vi "CurrentSweepExample.vi"(4 "Points":i32, 5 "milliseconds to wait":u32=10000, 6 "End Current":dbl=1.0, 7 "Start Current":dbl, 8 "Stanford Err":errorcluster, 9 "Stanford":refnum<visa-resource-name>, 10 "Keithley Err":errorcluster, 11 "Keithley":refnum<visa-resource-name>) -> (0 "Stanford Err Out":errorcluster, 1 "Stanford Out":refnum<visa-resource-name>, 2 "Keithley Err Out":errorcluster, 3 "Keithley Out":refnum<visa-resource-name>)   [LabVIEW 2013]
uses:
  <vilib>/Analysis/1siggen.llb/Ramp Pattern by Samples.vi
  Stop_B_Global.vi
  He3_Tlogger_Global 1.vi
  <vilib>/Analysis/NI_AALBase.lvlib
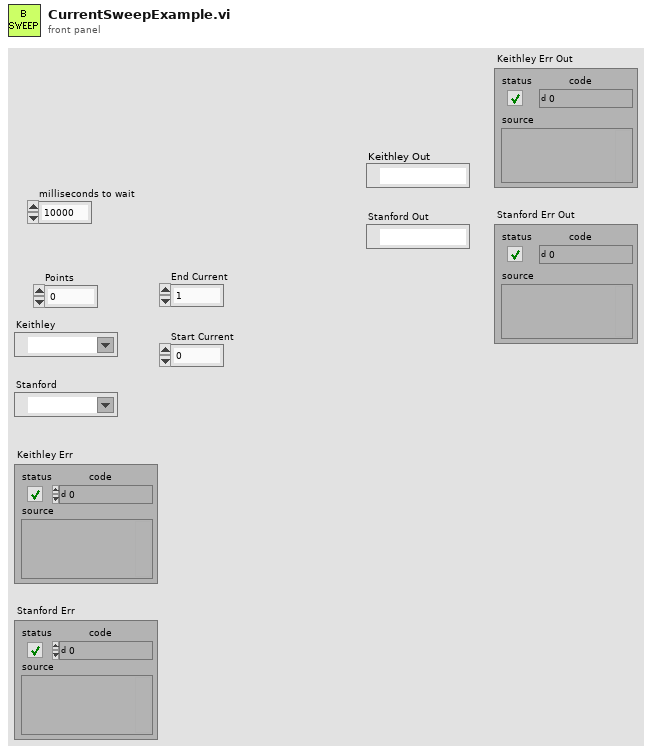
[diagram p1: front panel]
types:
  T1 = cluster{"Stanford Current":dbl, "X-Value":dbl, "Y-Value":dbl, "R-Value":dbl, "Theta-Value":dbl, "Reference Frequency":dbl, "Field":dbl, "Temperature":dbl, "Resistance":dbl, "Integration Time":dbl}
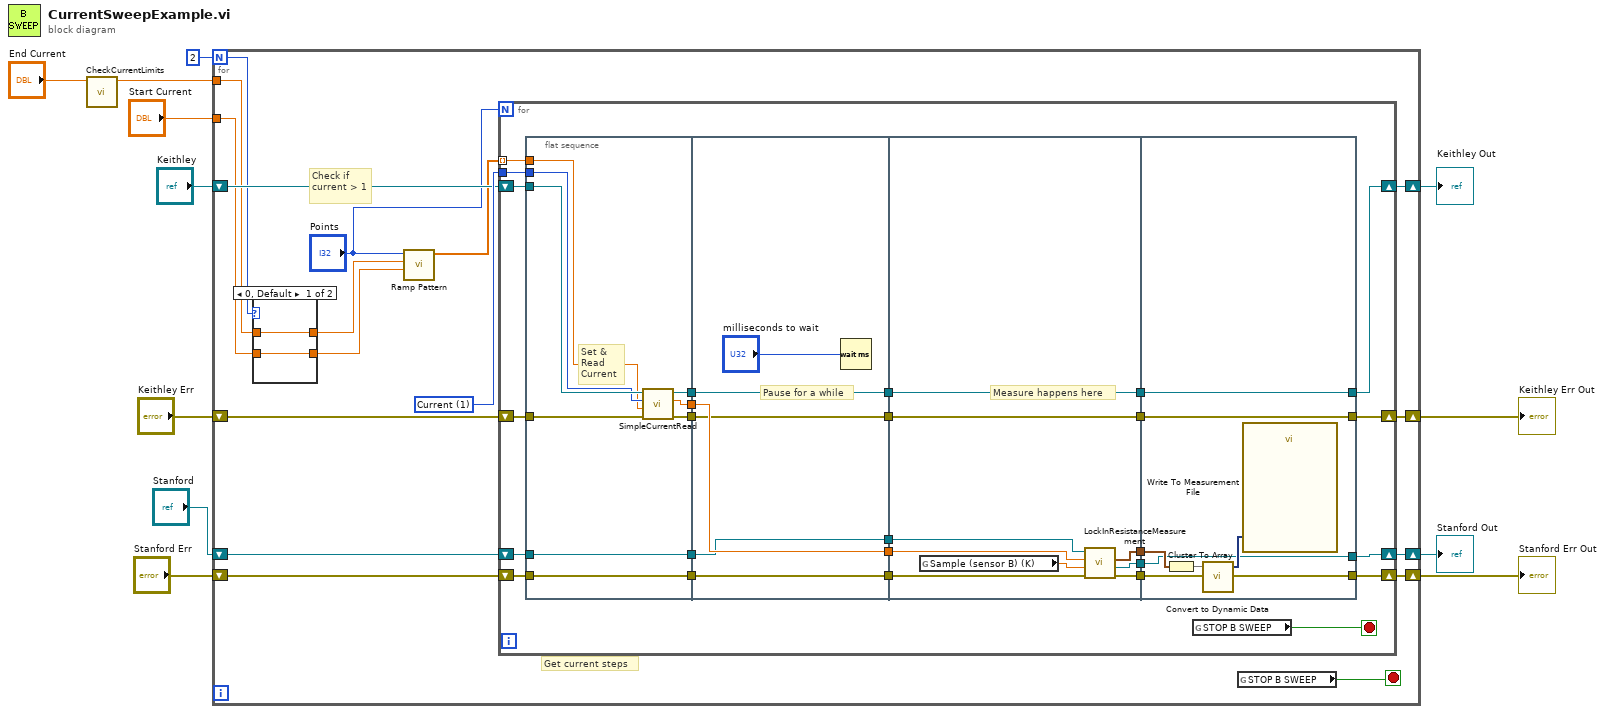
[diagram p0: block diagram]
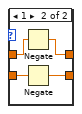
[diagram p2: hidden frame]
diagram:
  n1 = call "CheckCurrentLimits.vi"("End Current"="End Current") -> ("End Current"=w7:dbl)  [unwired: 10 in]
  n2 = for {
    N: 2 -> [w19]
    tunnel: w7 -> [w18]
    tunnel: "Start Current" -> [w17]
    shift-right: [w22] -> w1
    shift-left: "Keithley" -> [w28]
    shift-right: [w21] -> w2
    shift-left: "Keithley Err" -> [w27]
    shift-right: [w23] -> w3
    shift-left: "Stanford" -> [w25]
    shift-right: [w20] -> w4
    shift-left: "Stanford Err" -> [w14]
    stop <- w13 stop-if-true
    w29 = u16 1 items=["Volts", "Current", "Resistance"] ("Function (0: Volts)")
    # "Get current steps"
    # "Check if current > 1"
    n3 = case shown="0, Default" w19 {
      tunnel: w18 -> [w31 w33]
      tunnel: w17 -> [w30 w35]
      tunnel: [w30 w34] -> w16
      tunnel: [w31 w32] -> w15
      frame 0, Default {
      }
      frame 1 {
        n4 = Negate(x=w33) -> (-x=w32:dbl)
        n5 = Negate(x=w35) -> (-x=w34:dbl)
      }
    }
    n6 = call-poly <vilib>:"Ramp Pattern.vi"("start"=w16, "end"=w15, "samples"="Points") -> ("Ramp Pattern"=w26:dbl[])  [unwired: 7 in, 1 out]
    n7 = for {
      N: "Points" -> [_]
      tunnel: w29 -> [w61]
      tunnel: w26 -> [w58] mode=indexing
      shift-right: [w39] -> w23
      shift-left: w25 -> [w50]
      shift-right: [w47] -> w22
      shift-left: w28 -> [w60]
      shift-right: [w48] -> w21
      shift-left: w27 -> [w59]
      shift-right: [w37] -> w20
      shift-left: w14 -> [w45]
      stop <- w36 stop-if-true
      n8 = flat-sequence {
        tunnel: w61 -> [w67]
        tunnel: w60 -> [w68]
        tunnel: w59 -> [w65]
        tunnel: w58 -> [w66]
        tunnel: [w64] -> w57
        tunnel: [w63] -> w56
        tunnel: [w62] -> w55
        tunnel: [w70] -> w51
        tunnel: w50 -> [w70]
        tunnel: [w69] -> w46
        tunnel: w45 -> [w69]
        tunnel: w57 -> [w76]
        tunnel: w56 -> [w75]
        tunnel: w55 -> [w74]
        tunnel: [w76] -> w54
        tunnel: [w75] -> w53
        tunnel: [w74] -> w52
        tunnel: w51 -> [w72]
        tunnel: [w72] -> w49
        tunnel: w46 -> [w71]
        tunnel: [w71] -> w44
        tunnel: w54 -> [w85]
        tunnel: w53 -> [w80]
        tunnel: w52 -> [w84]
        tunnel: w49 -> [w83]
        tunnel: w44 -> [w82]
        tunnel: [w85] -> w43
        tunnel: [w84] -> w42
        tunnel: [w79] -> w41
        tunnel: [w78] -> w40
        tunnel: [w77] -> w38
        tunnel: [w91] -> w48
        tunnel: [w92] -> w47
        tunnel: w43 -> [w92]
        tunnel: w42 -> [w91]
        tunnel: w41 -> [w87]
        tunnel: w40 -> [w89]
        tunnel: [w87] -> w39
        tunnel: [w86] -> w37
        tunnel: w38 -> [w86]
        frame #0 {
          # "Set &\nRead\nCurrent"
          n9 = call "SimpleCurrentRead.vi"("error in (no error)"=w65, "Current Setting"=w66, "Function (0: Volts)"=w67, "Keithley In"=w68) -> ("error out"=w62:errorcluster, "Measured Current"=w63:dbl, "Keithley Out"=w64:refnum<visa-resource-name>)  [unwired: 5 in]
        }
        frame #1 {
          # "Pause for a while"
          n10 = Wait (ms)(milliseconds to wait="milliseconds to wait") -> ()  [unwired: 1 out]
        }
        frame #2 {
          # "Measure happens here"
          n11 = global read "He3_Tlogger_Global 1.vi" "Sample (sensor B) (K)"() -> (w81:dbl)
          n12 = call "LockInResistanceMeasurement.vi"("Stanford Error In"=w82, "Temperature"=w81, "Keithley Current"=w80, "Stanford ID"=w83) -> ("error out"=w77:errorcluster, "Stanford ID"=w79:refnum<visa-resource-name>, "output cluster"=w78:T1)  [unwired: 3 in, 1 out]
        }
        frame #3 {
          n13 = Cluster To Array(cluster=w89) -> (array=w88:dbl[])
          n14 = call "Convert to Dynamic Data"("Array"=w88) -> ("Dynamic Data Type"=w90:dynamicdata)  [unwired: 3 in]
          n15 = call "Write To Measurement File"("Signals"=w90) -> ()  [unwired: 16 in, 3 out]
        }
      }
      n16 = global read "Stop_B_Global.vi" "STOP B SWEEP"() -> (w36:bool)
    }
    n17 = global read "Stop_B_Global.vi" "STOP B SWEEP"() -> (w13:bool)
  }
  "Keithley Out" <- w1
  "Stanford Out" <- w3
  "Stanford Err Out" <- w4
  "Keithley Err Out" <- w2
